vi "Rotate Object.vi"(8 "error in (no error)":errorcluster, 9 "Angle":sgl, 10 "Axis":cluster{"X":sgl, "Y":sgl, "Z":sgl}, 11 "Scene.Object In":refnum<vi>) -> (0 "error out":errorcluster, 3 "Scene.Object Out":refnum<vi>)   [LabVIEW 2017, in "NI_3D Picture Control.lvlib"]
doc: "Rotates an object in a 3D scene by the values <B>Axis</B> and <B>Angle</B>. This VI performs a relative rotation from the object's current position."
uses:
  <vilib>/picture/3D Picture Control/NI_3D Picture Control.lvlib
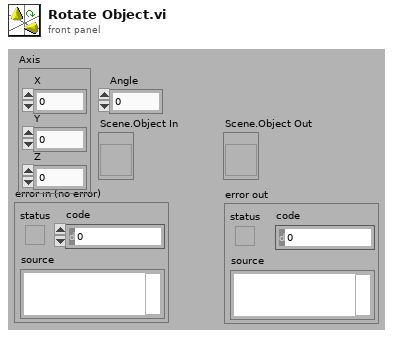
[diagram p1: front panel]
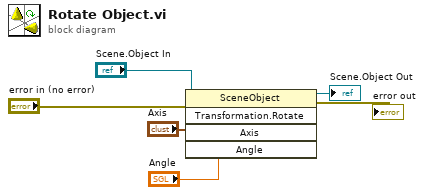
[diagram p0: block diagram]
diagram:
  n1 = invoke class="SceneObject" method="Transformation.Rotate"(reference="Scene.Object In", error in="error in (no error)", "Axis"="Axis", "Angle"="Angle") -> (reference out=→"Scene.Object Out":refnum<vi>, error out=→"error out":errorcluster)  [unwired: 1 in, 3 out]
